vi "Set Message Name.vi"(8 "error in":errorcluster, 10 "message name":string, 11 "message in":T1 format="%.0x") -> (0 "error out":errorcluster, 3 "message out":T1 format="%.0x")   [LabVIEW 2020, in "Ballard MIL-STD-1553 Scripting.lvlib"]
doc: "Reads the <b>description</b> field of the input <b>Ballard MIL-STD 1553 custom device</b>."
uses:
  <vilib>/NI VeriStand/Custom Device API/Custom Device Item Ref.ctl
  Constants.vi
  Ballard MIL-STD-1553 Scripting.lvlib
  <vilib>/NI VeriStand/Custom Device API/Custom Device API.lvlib
  <vilib>/NI VeriStand/Custom Device API/Set Item Property (String).vi
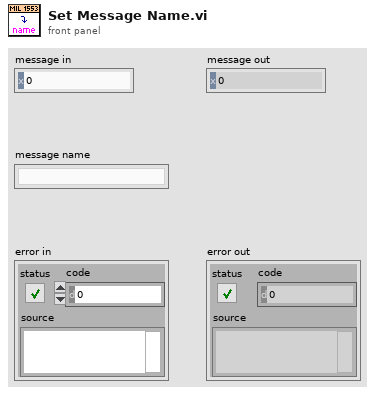
[diagram p1: front panel]
types:
  T1 = typedef "Custom Device API.lvlib/Custom Device Item Ref.ctl" = u64
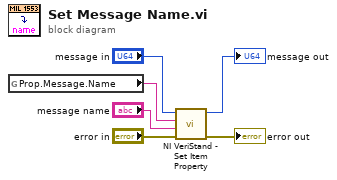
[diagram p0: block diagram]
diagram:
  n1 = global read "Constants.vi" "Prop.Message.Name"() -> (w2:string)
  n2 = call-poly <vilib>:"NI VeriStand - Set Item Property.vi"("error in (no error)"="error in", "Value"="message name", "Property Name"=w2, "Item Ref in"="message in") -> ("error out"=→"error out":errorcluster, "Item Ref out"=→"message out":T1)  [unwired: 5 in, 1 out]
